vi "Read Latest Value.vi"(8 "error in (no error)":errorcluster, 11 "Ring buffer DVR in":refnum<data-value>) -> (0 "error out":errorcluster, 1 "Values":u8[](array[numeric]), 2 "Timestamp":u64, 3 "Ring buffer DVR out":refnum<data-value>, 4 "empty buffer?":bool)   [LabVIEW 2021, in "Ring Buffer Time Series Data.lvlib"]
uses:
  Ring Buffer Time Series Data.lvlib
  SubVIs/DVR data.ctl
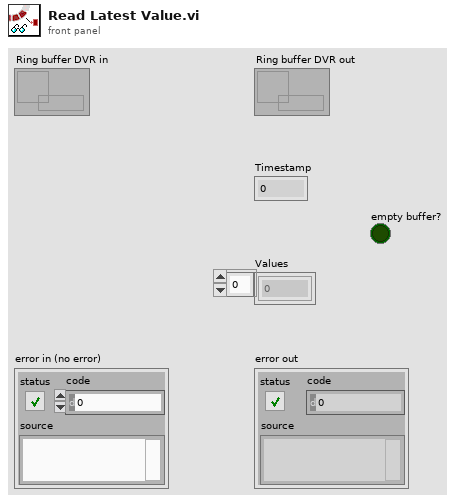
[diagram p1: front panel]
types:
  T1 = typedef "Ring Buffer Time Series Data.lvlib/DVR data.ctl" = cluster{"Timestamps":u64[], "Values":u8[], "#bytes per timestamp":i32, "Index":i32, "Size (#timestamps)":i32, "Full?":bool}
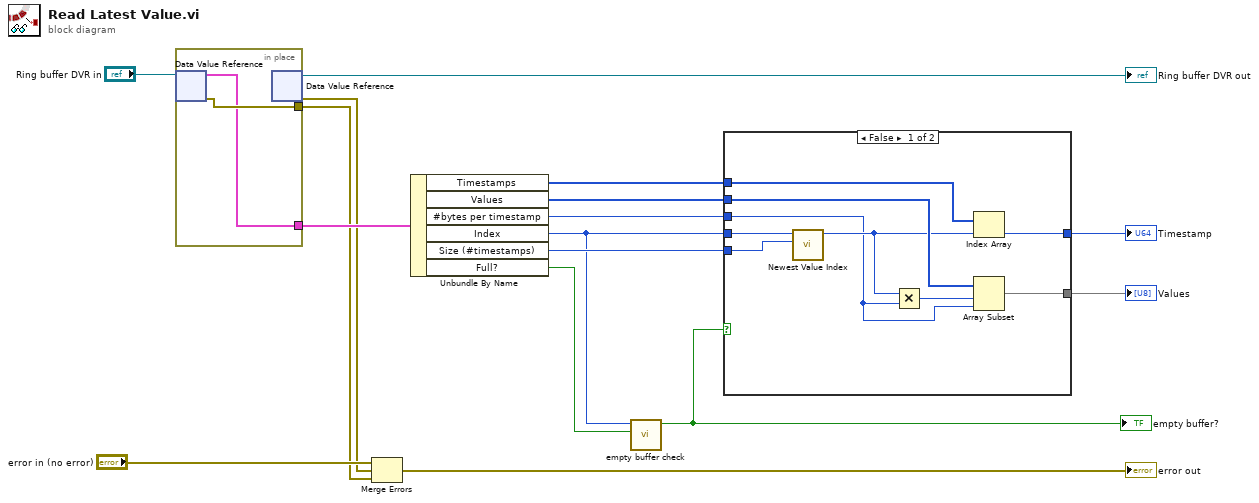
[diagram p0: block diagram]
diagram:
  n1 = in-place {
    in-place-border: [w18] -> w4
    in-place-border: [w17] -> w10
    n2 = in-place-dvr #1("Ring buffer DVR in") -> (w17:T1, w18:errorcluster)
    n3 = in-place-dvr #1() -> (→"Ring buffer DVR out":refnum<data-value>, w5:errorcluster)  [unwired: 1 in]
  }
  n4 = Merge Errors("error in (no error)", w5, w4) -> (→"error out":errorcluster)
  n5 = Unbundle By Name(w10) -> ("Timestamps"=w9:u64[], "Values"=w8:u8[], "#bytes per timestamp"=w6:i32, "Index"=w3:i32, "Size (#timestamps)"=w7:i32, "Full?"=w2:bool)
  n6 = call "empty buffer check.vi"("Full?"=w2, "Index"=w3) -> ("empty buffer?"=w1:bool)  [unwired: 9 in]
  "empty buffer?" <- w1
  n7 = case shown="False" w1 {
    tunnel: [w27 _] -> w14
    tunnel: [w26 _] -> w13
    tunnel: w9 -> [w25 _]
    tunnel: w8 -> [w24 _]
    tunnel: w7 -> [w21 _]
    tunnel: w6 -> [w20 _]
    tunnel: w3 -> [w19 _]
    frame False {
      n8 = call "Newest Value Index.vi"("Size"=w21, "Index"=w19) -> ("Newest value index"=w22:i32)  [unwired: 9 in]
      n9 = Multiply(x=w22, y=w20) -> (x*y=w23:i32)
      n10 = Index Array(array=w25, index=w22) -> (element=w26:u64)
      n11 = Array Subset(array=w24, index=w23, length=w20) -> (w27:u8[])
    }
    frame True {
    }
  }
  "Timestamp" <- w13
  "Values" <- w14
